vi "GUI_laptop v8.vi"() -> ()   [LabVIEW 2019]
uses:
  <vilib>/Math Plots/3D Math Plots/3D Scatter/3D Scatter XCtrl/3D Scatter.xctl
  <vilib>/Platform/TimedLoop/XDataNode/timing_clust.ctl
  <vilib>/Platform/TimedLoop/XDataNode/nitl_modes.ctl
  <vilib>/Platform/TimedLoop/XDataNode/wakeup.ctl
  <vilib>/Analysis/_algsub.llb/Real Vector Norm.vi
  <vilib>/Instr/_visa.llb/VISA Configure Serial Port (Instr).vi
  <vilib>/Utility/file.llb/Write Delimited Spreadsheet (DBL).vi
  <vilib>/Math Plots/3D Math Plots/3D Scatter/3D Scatter Datatype/Public/Plot Helper (Vector).vi
  <vilib>/platform/TimedLoop/XDataNode/XDataNode.xnode
  <vilib>/Platform/TimedLoop/XDataNode/XDNodeRunTimeDep.lvlib
  <vilib>/Analysis/NI_AALPro.lvlib
  <vilib>/Math Plots/3D Math Plots/3D Scatter/3D Scatter Datatype/3D Scatter Datatype.lvclass
panel:
  out "send values":dbl[](array[numeric])
  out "Robot Feedback (xyz)":dbl[](array[numeric])
  in  "UDP Send":bool
  in  "UDP Recv":bool
  in  "L5 bound":dbl=1000.0
  in  "L4 bound (deg)":dbl=1000.0
  in  "L3 bound (mm)":dbl=1000.0
  in  "L2 bound (deg)":dbl=1000.0
  in  "L1 bound (deg)":dbl=1000.0
  in  "Joystick Type":dbl(ring) items=["Rigid Joystick", "Free Joystick"]
  out "Finished Late? [i-1]":bool
  in  "Epsilon":dbl=0.2
  out "3D Scatter":refnum<class "3D Plot Datatype.lvclass">[](xcontrol)
  out "Random Point":dbl[](array[numeric])
  out "Virtual Cursor":dbl[](array[numeric])
  out "Iteration Duration":i64
  in  "Num of Points":i32=10
  in  "z bound":dbl=2.0
  in  "y bound":dbl=5.0
  in  "x bound":dbl=5.0
  in  "Stop":bool
  in  "Round Decimals":dbl=2.0 format="%#_15g"
  in  "Save  Data":bool
  in  "Save Path":path
  in  "x speed":dbl=0.5
  in  "z speed":dbl=0.5
  in  "y speed":dbl=0.5
  out "error out":errorcluster
  in  "baud rate":u32=115200
  in  "VISA resource name":refnum<visa-resource-name>
  # "TODO: fix the bounds; currently bounds are arbitrary"
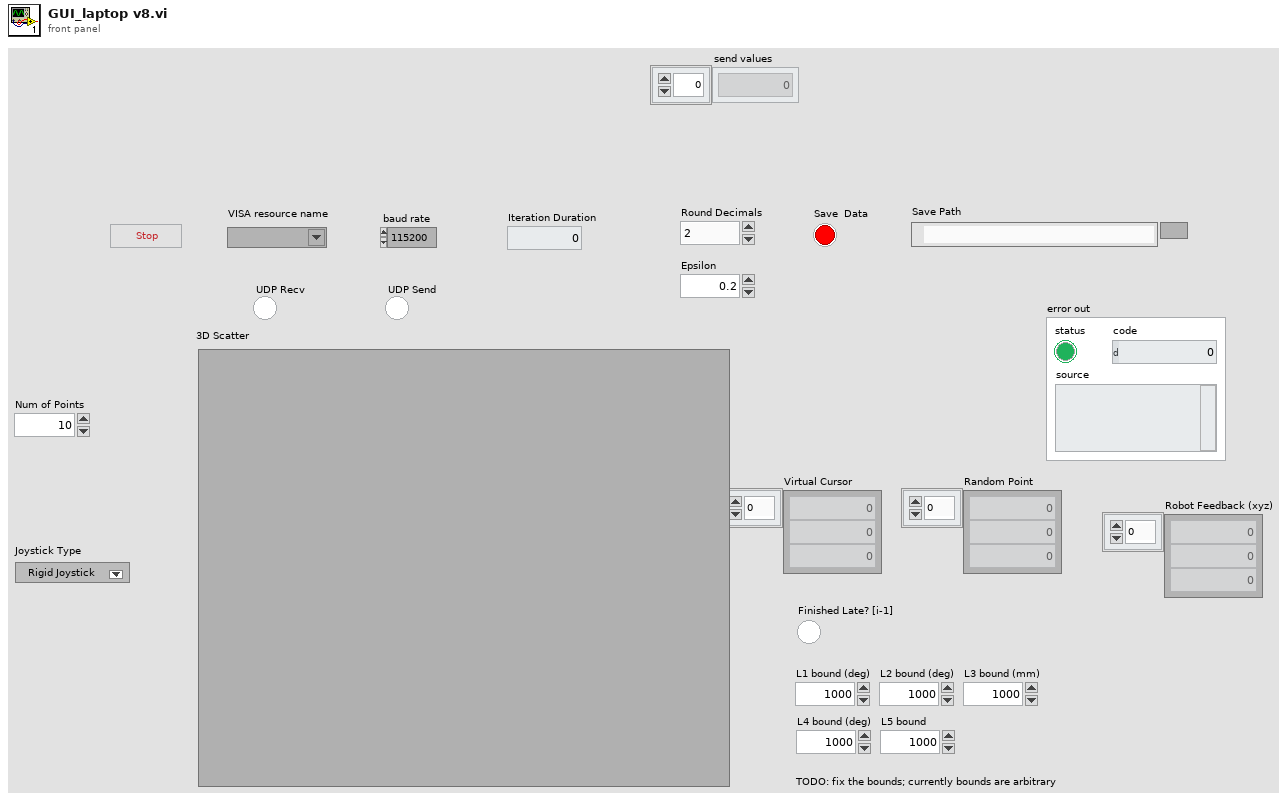
[diagram p1: front panel]
types:
  T1 = typedef "XDNodeRunTimeDep.lvlib/timing_clust.ctl" = cluster{"Expected End [f-1]":u64, "Actual End [f-1]":u64, "Finished Late? [f-1]":bool, "Expected End [i-1]":u64, "Actual End [i-1]":u64, "Finished Late? [i-1]":bool, "Expected Start [i]":u64, "Actual Start [i]":u64, "Expected Start [f]":u64, "Actual Start [f]":u64, "Source Name":string, "Structure Name":string, "Period":i64, "Deadline":i64, "Offset":i64, "Start":i64, "Priority":i32, "Timeout":i32, "Mode":T2, "Wakeup Reason":T3, "Error":errorcluster, "Source Type":string, "Secondary Source Type":string, "Global End Time":u64, "Global Start Time":u64, "Frame Duration":u64, "Iteration Duration":u64, "Assigned CPU":i32, "I/O Scan Engine Mode":u32}
  T2 = typedef "XDNodeRunTimeDep.lvlib/nitl_modes.ctl" = enum32{"No Change", "Process missed periods, maintain original phase", "Discard missed periods, maintain original phase", "Process missed periods, ignore original phase", "Discard missed periods, ignore original phase"}
  T3 = typedef "XDNodeRunTimeDep.lvlib/wakeup.ctl" = enum32{"Normal", "Aborted", "Asynchronous wakeup", "Timing source error", "Timed loop error", "Timeout"}
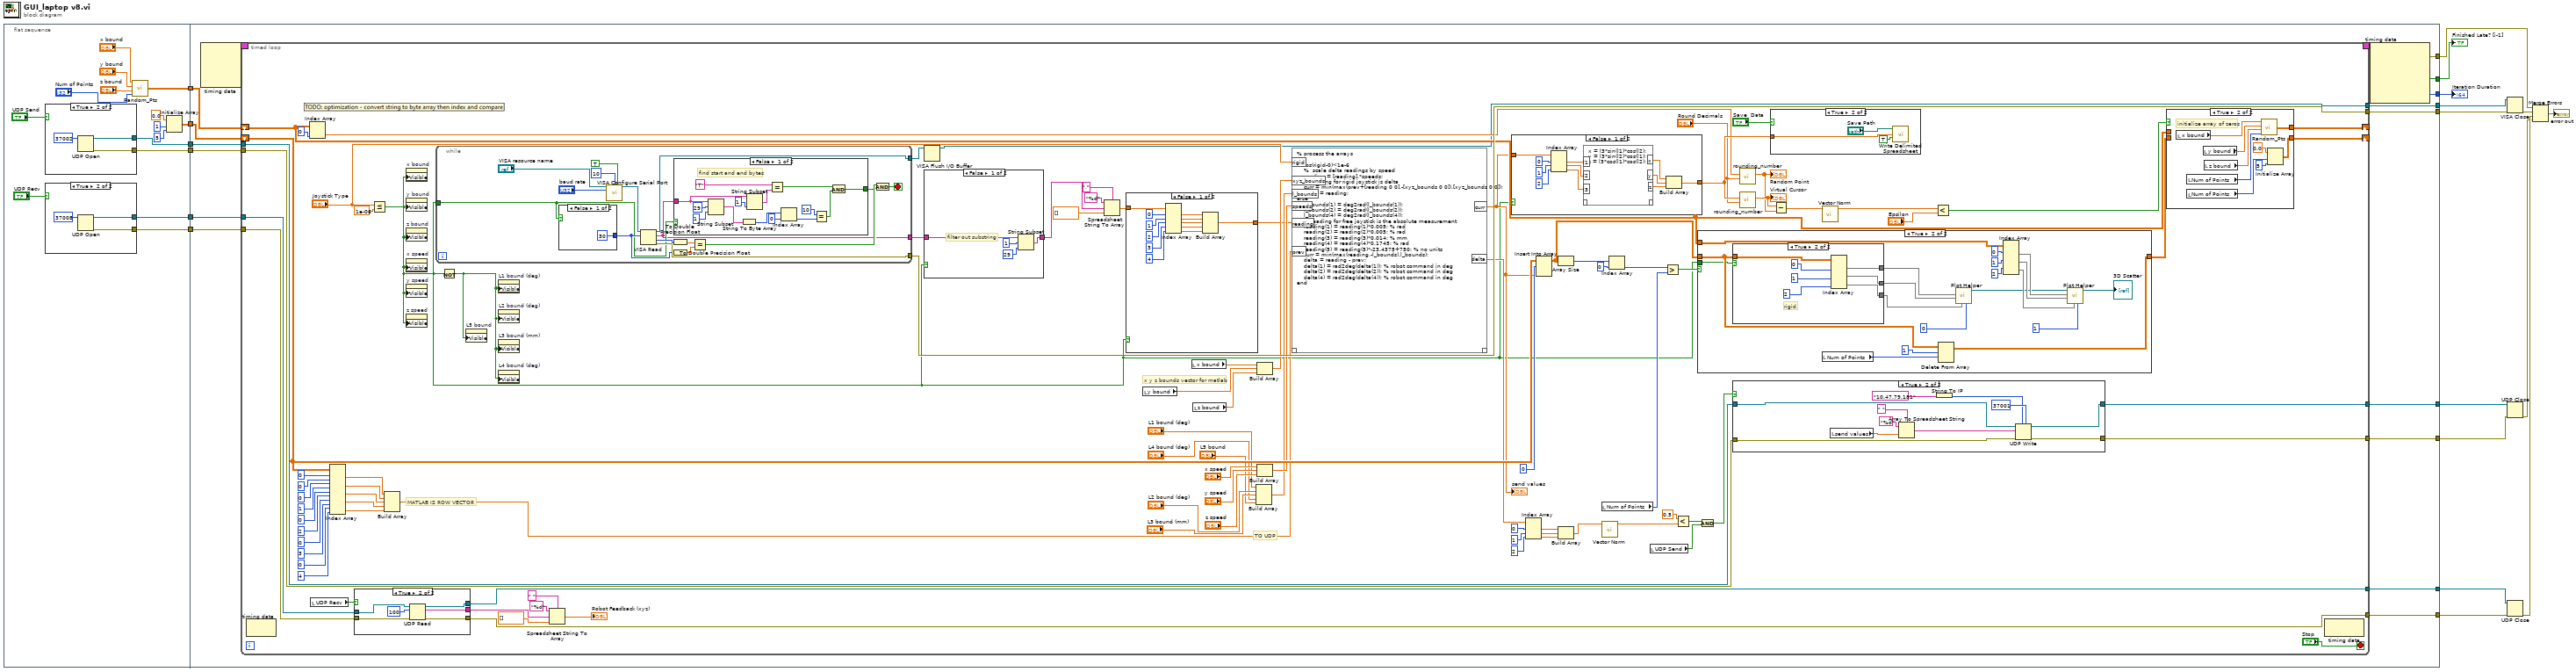
[diagram p0: block diagram]
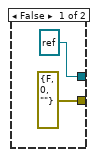
[diagram p2: hidden frame]
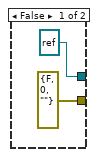
[diagram p3: hidden frame]
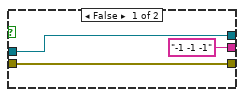
[diagram p5: hidden frame]
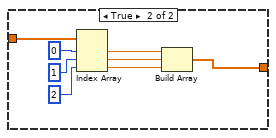
[diagram p9: hidden frame]
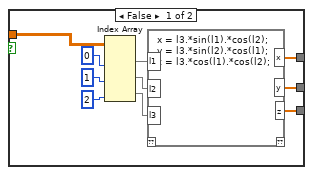
[diagram p12: hidden frame]
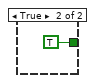
[diagram p13: hidden frame]
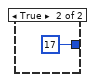
[diagram p14: hidden frame]
diagram:
  n1 = flat-sequence {
    tunnel: [w26] -> w15
    tunnel: [w30] -> w14
    tunnel: [w25] -> w13
    tunnel: [w24] -> w12
    tunnel: [w21] -> w11
    tunnel: [w20] -> w10
    tunnel: [w59] -> w19
    tunnel: [w58] -> w18
    tunnel: [w56] -> w9
    tunnel: [w54] -> w17
    tunnel: [w53] -> w16
    tunnel: w15 -> [w57]
    tunnel: w14 -> [w55]
    tunnel: w13 -> [w52]
    tunnel: w12 -> [w51]
    tunnel: w11 -> [w50]
    tunnel: w10 -> [w49]
    tunnel: [w48] -> w3
    tunnel: [w47] -> w8
    tunnel: [w46] -> w2
    tunnel: [w45] -> w1
    frame #0 {
      n2 = case shown="True" "UDP Send" {
        tunnel: [refnum<k16> refnum ("port") w38] -> w25
        tunnel: [errorcluster {"status"=FALSE, "code"=0, "source"=""} ("error out") w37] -> w20
        frame False {
        }
        frame True {
          n3 = UDP Open(11:u16 37002 ("port")) -> (port=w38:refnum<k16>, 0:w37:errorcluster)  [unwired: 4 in, 1 out]
        }
      }
      n4 = case shown="True" "UDP Recv" {
        tunnel: [refnum<k16> refnum ("port") w43] -> w24
        tunnel: [errorcluster {"status"=FALSE, "code"=0, "source"=""} ("error out") w42] -> w21
        frame False {
        }
        frame True {
          n5 = UDP Open(11:u16 37008 ("port")) -> (port=w43:refnum<k16>, 0:w42:errorcluster)  [unwired: 4 in, 1 out]
        }
      }
      n6 = call "Random_Pts.vi"("Num of Points"="Num of Points", "z bound"="z bound", "y bound"="y bound", "x bound"="x bound") -> ("appended array"=w30:dbl[][])
      n7 = Initialize Array(0.0 ("element"), 1 ("dimension size"), 5 ("dimension size")) -> (w26:dbl[][])
    }
    frame #1 {
      n8 = node-c288() -> (w61:T1)  [unwired: 4 in]
      n9 = timed-loop {
        tunnel: [w92] -> w59
        tunnel: [w156] -> w58
        shift-right: [w155] -> _
        shift-left: w57 -> [w154]
        timing: w61 -> [_]
        timing-out: [_] -> w60
        shift-right: [w150] -> _
        shift-left: w55 -> [w151]
        tunnel: w52 -> [w91]
        tunnel: w51 -> [w90]
        tunnel: w50 -> [w88]
        tunnel: w49 -> [w87]
        tunnel: [w86] -> w48
        tunnel: [w85] -> w47
        tunnel: [w84] -> w46
        tunnel: [w83] -> w45
        stop <- "Stop" stop-if-true
        # "TO UDP"
        # "MATLAB IS ROW VECTOR"
        # "x y z bounds vector for matlab"
        n10 = node-c288() -> ()  [unwired: 1 in, 1 out]
        n11 = Index Array(array=w151, index (col)=0 ("index (row)")) -> (element=w103:dbl[])  [unwired: 1 in]
        n12 = local read "UDP Recv"() -> (w89:bool)
        n13 = Index Array(array=w154, index (row) #1=0 ("disabled index (row)"), index (col) #1=0 ("disabled index (col)"), index (row) #2=0 ("disabled index (row)"), index (col) #2=1 ("disabled index (col)"), index (row) #3=0 ("disabled index (row)"), index (col) #3=2 ("disabled index (col)"), index (row) #4=0 ("disabled index (row)"), index (col) #4=3 ("disabled index (col)"), index (row) #5=0 ("disabled index (row)"), index (col) #5=4 ("disabled index (col)")) -> (element #1=w127:dbl, element #2=w126:dbl, element #3=w125:dbl, element #4=w111:dbl, element #5=w110:dbl)
        n14 = case shown="True" w89 {
          tunnel: w90 -> [w172 w179]
          tunnel: w88 -> [w173 w178]
          tunnel: [w173 w177] -> w86
          tunnel: [w172 w176] -> w84
          tunnel: ["-1 -1 -1" w174] -> w79
          frame False {
          }
          frame True {
            n15 = UDP Read(connection ID=w179, max size (548)=100, 8:w178) -> (data out=w174:string, error out=w177:errorcluster, 3:w176:refnum<k16>)  [unwired: 1 in, 2 out]
          }
        }
        n16 = Less Or Equal?(x="Joystick Type", y=1e-06) -> (x <= y?=w63:bool)
        n17 = Build Array(w127, w126, w125, w111, w110) -> (w124:dbl[])
        n18 = property on="x bound" class="DigNum (strict)"("Visible"=w63) -> ()  [unwired: 2 in, 2 out]
        n19 = property on="y bound" class="DigNum (strict)"("Visible"=w63) -> ()  [unwired: 2 in, 2 out]
        n20 = property on="z bound" class="DigNum (strict)"("Visible"=w63) -> ()  [unwired: 2 in, 2 out]
        n21 = property on="x speed" class="DigNum (strict)"("Visible"=w63) -> ()  [unwired: 2 in, 2 out]
        n22 = property on="y speed" class="DigNum (strict)"("Visible"=w63) -> ()  [unwired: 2 in, 2 out]
        n23 = property on="z speed" class="DigNum (strict)"("Visible"=w63) -> ()  [unwired: 2 in, 2 out]
        n24 = while {
          tunnel: [w268] -> w105
          tunnel: [w281] -> w156
          tunnel: [w275] -> w93
          tunnel: w63 -> [w269]
          stop <- w271 stop-if-true
          n25 = case shown="False" w269 {
            tunnel: [30 u32 17 ("byte count")] -> w274
            frame False {
            }
            frame True {
            }
          }
          n26 = call-poly "VISA Configure Serial Port"("VISA resource name"="VISA resource name", "termination char\n(0xA = '\\n' = LF)"=u8 10 ("termination char\n(0xA = '\\n' = LF)"), "Enable Termination\nChar (T)"=TRUE ("Enable Termination\nChar (T)"), "baud rate (9600)"="baud rate") -> ("VISA resource name out"=w276:refnum<visa-resource-name>)  [unwired: 10 in, 1 out]
          n27 = VISA Read(VISA resource name=w276, byte count=w274) -> (VISA resource name out=w275:refnum<visa-resource-name>, read buffer=w268:string, return count=w283:u32, error out=w281:errorcluster)  [unwired: 1 in]
          n28 = To Double Precision Float(number=w283) -> (double precision float=w282:dbl)
          n29 = To Double Precision Float(number=w274) -> (double precision float=w273:dbl)
          n30 = case shown="False" w269 {
            tunnel: [w290 TRUE] -> w270
            tunnel: w268 -> [w293 _]
            frame False {
              # "find start and end bytes"
              n31 = String Subset(string=w293, offset (0)=29, length (rest)=1) -> (substring=w288:string)
              n32 = String To Byte Array(string=w288) -> (unsigned byte array=w287:u8[])
              n33 = String Subset(string=w293, length (rest)=1) -> (substring=w296:string)  [unwired: 1 in]
              n34 = Equal?(x="T", y=w296) -> (x = y?=w292:bool)
              n35 = Index Array(array=w287, index=0) -> (element=w285:u8)
              n36 = Equal?(x=10, y=w285) -> (x = y?=w291:bool)
              n37 = And(x=w292, y=w291) -> (x .and. y?=w290:bool)
            }
            frame True {
            }
          }
          n38 = Equal?(x=w282, y=w273) -> (x = y?=w272:bool)
          n39 = And(x=w272, y=w270) -> (x .and. y?=w271:bool)
        }
        n40 = Not(x=w63) -> (.not. x?=w62:bool)
        n41 = property on="L5 bound" class="DigNum (strict)"("Visible"=w62) -> ()  [unwired: 2 in, 2 out]
        n42 = property on="L1 bound (deg)" class="DigNum (strict)"("Visible"=w62) -> ()  [unwired: 2 in, 2 out]
        n43 = property on="L2 bound (deg)" class="DigNum (strict)"("Visible"=w62) -> ()  [unwired: 2 in, 2 out]
        n44 = property on="L3 bound (mm)" class="DigNum (strict)"("Visible"=w62) -> ()  [unwired: 2 in, 2 out]
        n45 = property on="L4 bound (deg)" class="DigNum (strict)"("Visible"=w62) -> ()  [unwired: 2 in, 2 out]
        n46 = Spreadsheet String To Array(delimiter (Tab)=" ", format string="%d", spreadsheet string=w79, array type (2D Dbl)=dbl[] []) -> (array=→"Robot Feedback (xyz)":dbl[])
        n47 = VISA Flush I/O Buffer(VISA resource name=w93) -> (VISA resource name out=w92:refnum<visa-resource-name>)  [unwired: 2 in, 1 out]
        n48 = case shown="False" w63 {
          tunnel: w105 -> [w197 w198]
          tunnel: [w194 w198] -> w104
          frame False {
            # "filter out substring"
            n49 = String Subset(string=w197, offset (0)=1, length (rest)=29) -> (substring=w194:string)
          }
          frame True {
          }
        }
        n50 = Spreadsheet String To Array(delimiter (Tab)=",", format string="%d", spreadsheet string=w104, array type (2D Dbl)=dbl[] []) -> (array=w107:dbl[])
        n51 = case shown="False" w63 {
          tunnel: w107 -> [w199 w212]
          tunnel: [w204 w211] -> w106
          frame False {
            n52 = Index Array(array=w199, index #1=0 ("Plot ID"), index #2=1 ("Plot ID"), index #3=2 ("Plot ID"), index #4=3 ("Plot ID"), index #5=4 ("Plot ID")) -> (element #1=w207:dbl, element #2=w206:dbl, element #3=w205:dbl, element #4=w201:dbl, element #5=w200:dbl)
            n53 = Build Array(w207, w206, w205, w201, w200) -> (w204:dbl[])
          }
          frame True {
            n54 = Index Array(array=w212, index #1=0 ("Plot ID"), index #2=1 ("Plot ID"), index #3=2 ("Plot ID")) -> (element #1=w215:dbl, element #2=w214:dbl, element #3=w213:dbl)
            n55 = Build Array(w215, w214, w213) -> (w211:dbl[])
          }
        }
        n56 = local read "y bound"() -> (w129:dbl)
        n57 = local read "x bound"() -> (w130:dbl)
        n58 = local read "z bound"() -> (w128:dbl)
        n59 = Build Array("L1 bound (deg)", "L2 bound (deg)", "L3 bound (mm)", "L4 bound (deg)", "L5 bound") -> (w118:dbl[])
        n60 = Build Array(w130, w129, w128) -> (w122:dbl[])
        n61 = Build Array("x speed", "y speed", "z speed") -> (w123:dbl[])
        n62 = script code="% process the arrays\n\nif abs(rigid-0)<1e-6\n    %  scale delta readings by speed\n    reading = [reading].*speeds;\n    % reading for rigid joystick is delta\n    curr = min(max(prev+[reading 0 0],-[xyz_bounds 0 0]),[xyz_bounds 0 0]);\n    delta = reading;\nelse\n    l_bounds(1) = deg2rad(l_bounds(1));\n    l_bounds(2) = deg2rad(l_bounds(2));\n    l_bounds(4) = deg2rad(l_bounds(4));\n    % reading for free joystick is the absolute measurement\n    reading(1) = reading(1)*0.005; % rad\n    reading(2) = reading(2)*0.005; % rad\n    reading(3) = reading(3)*0.014; % mm\n    reading(4) = reading(4)*0.1745; % rad\n    reading(5) = reading(5)*-23.4375+750; % no units\n    curr = min(max(reading,-l_bounds),l_bounds);\n    delta = reading - prev;\n    delta(1) = rad2deg(delta(1)); % robot command in deg\n    delta(2) = rad2deg(delta(2)); % robot command in deg\n    delta(4) = rad2deg(delta(4)); % robot command in deg\nend"("xyz_bounds"=w122, "speeds"=w123, "reading"=w106, "prev"=w124, "rigid"="Joystick Type", "l_bounds"=w118) -> ("curr"=w64:dbl[], "delta"=w72:dbl[])  [unwired: 1 in, 1 out]
        "send values" <- w64
        n63 = case shown="False" w63 {
          tunnel: w64 -> [w226 w230]
          tunnel: [w219 w230] -> w152
          frame False {
            n64 = Index Array(array=w226, index #1=0 ("Plot ID"), index #2=1 ("Plot ID"), index #3=2 ("Plot ID")) -> (element #1=w225:dbl, element #2=w224:dbl, element #3=w223:dbl)
            n65 = script code="x = l3*sin(l1)*cos(l2);\ny = l3*sin(l2)*cos(l1);\nz = l3*cos(l1)*cos(l2);"("l1"=w225, "l2"=w224, "l3"=w223) -> ("x"=w222:dbl, "y"=w221:dbl, "z"=w220:dbl)  [unwired: 1 in, 1 out]
            n66 = Build Array(w222, w221, w220) -> (w219:dbl[])
          }
          frame True {
          }
        }
        n67 = Index Array(array=w72, index #1=0 ("disabled index (col)"), index #2=1 ("disabled index (col)"), index #3=2 ("disabled index (col)")) -> (element #1=w68:dbl, element #2=w67:dbl, element #3=w66:dbl)
        n68 = Insert Into Array(array=w154, index (row)=0, new element=w64) -> (w135:dbl[][])  [unwired: 1 in]
        n69 = Array Size(array=w135) -> (size(s)=w137:i32[])
        n70 = Build Array(w68, w67, w66) -> (w65:dbl[])
        n71 = local read "Num of Points"() -> (w136:i32)
        n72 = call-poly <vilib>:"Vector Norm.vi"("Input Vector"=w65) -> ("norm"=w77:dbl)  [unwired: 9 in, 1 out]
        n73 = Index Array(array=w137, index=0) -> (element=w138:i32)
        n74 = local read "UDP Send"() -> (w74:bool)
        n75 = Greater?(x=w138, y=w136) -> (0:w134:bool)
        n76 = Less?(x=0.5, y=w77) -> (x < y?=w75:bool)
        n77 = case shown="True" w134 {
          tunnel: w135 -> [w231 w249]
          tunnel: [w231 w248] -> w153
          tunnel: w151 -> [_ w247]
          tunnel: w63 -> [_ w232]
          frame False {
          }
          frame True {
            n78 = case shown="True" w232 {
              tunnel: w249 -> [w260 w264]
              tunnel: [w251 w263] -> w238
              tunnel: [w252 w262] -> w237
              tunnel: [w253 w261] -> w236
              frame False {
                n79 = Index Array(array=w260, index (col) #1=0 ("Plot ID"), index (col) #2=1 ("Plot ID"), index (col) #3=2 ("Plot ID")) -> (element #1=w256:dbl[], element #2=w255:dbl[], element #3=w254:dbl[])  [unwired: 3 in]
                n80 = script code="x = l3.*sin(l1).*cos(l2);\ny = l3.*sin(l2).*cos(l1);\nz = l3.*cos(l1).*cos(l2);"("l1"=w256, "l2"=w255, "l3"=w254) -> ("x"=w251:dbl[], "y"=w252:dbl[], "z"=w253:dbl[])  [unwired: 1 in, 1 out]
              }
              frame True {
                # "rigid"
                n81 = Index Array(array=w264, index (col) #1=0 ("disabled index (col)"), index (col) #2=1 ("index (col)"), index (col) #3=2 ("index (col)")) -> (element #1=w263:dbl[], element #2=w262:dbl[], element #3=w261:dbl[])  [unwired: 3 in]
              }
            }
            n82 = local read "Num of Points"() -> (w246:i32)
            n83 = Delete From Array(array=w249, length=1, index (row)=w246) -> (array with subset deleted=w248:dbl[][])  [unwired: 1 in, 1 out]
            n84 = call-poly <vilib>:"Plot Helper.vi"("Plot ID"=0, "z vector"=w236, "y vector"=w237, "x vector"=w238) -> ("3D Plot lvclass Array out"=w240:refnum<class "3D Plot Datatype.lvclass">[])  [unwired: 2 in, 5 out]
            n85 = Index Array(array=w247, index (row) #1=0 ("index (row)"), index (row) #2=1 ("index (row)"), index (row) #3=2 ("index (row)")) -> (element #1=w244:dbl[], element #2=w243:dbl[], element #3=w242:dbl[])  [unwired: 3 in]
            n86 = call-poly <vilib>:"Plot Helper.vi"("Plot ID"=1, "z vector"=w242, "y vector"=w243, "x vector"=w244, "3D Plot lvclass Array in"=w240) -> ("3D Plot lvclass Array out"=→"3D Scatter":refnum<class "3D Plot Datatype.lvclass">[])  [unwired: 1 in, 5 out]
          }
        }
        n87 = And(x=w75, y=w74) -> (x .and. y?=w73:bool)
        n88 = case shown="True" w73 {
          tunnel: w91 -> [w158 w170]
          tunnel: w87 -> [w159 w166]
          tunnel: [w159 w162] -> w85
          tunnel: [w158 w161] -> w83
          frame False {
          }
          frame True {
            n89 = local read "send values"() -> (w160:dbl[])
            n90 = Array To Spreadsheet String(delimiter (Tab)=" ", array=w160, 3:"%d" ("format string")) -> (spreadsheet string=w167:string)
            n91 = String To IP(1:"10.47.79.181" ("name")) -> (0:w164:u32)
            n92 = UDP Write(address=w164, port or service name=u16 37001, connection ID=w170, data in=w167, 8:w166) -> (error out=w162:errorcluster, 3:w161:refnum<k16>)  [unwired: 1 in]
          }
        }
        n93 = call "rounding_number.vi"("power of ten"="Round Decimals", "Array"=w103) -> ("rounded"=w99:dbl[])  [unwired: 9 in]
        "Random Point" <- w99
        n94 = call "rounding_number.vi"("power of ten"="Round Decimals", "Array"=w152) -> ("rounded"=w100:dbl[])  [unwired: 9 in]
        "Virtual Cursor" <- w100
        n95 = case shown="True" "Save  Data" {
          tunnel: w152 -> [_ w180]
          frame False {
          }
          frame True {
            n96 = call-poly <vilib>:"Write Delimited Spreadsheet.vi"("file path (dialog if empty)"="Save Path", "1D data"=w180, "append to file? (new file:F)"=TRUE) -> ()  [unwired: 11 in, 2 out]
          }
        }
        n97 = Subtract(x=w100, y=w99) -> (x-y=w98:dbl[])
        n98 = call-poly <vilib>:"Vector Norm.vi"("Input Vector"=w98) -> ("norm"=w97:dbl)  [unwired: 9 in, 1 out]
        n99 = Less?(x=w97, y="Epsilon") -> (x < y?=w95:bool)
        n100 = case shown="True" w95 {
          tunnel: w151 -> [w184 _]
          tunnel: [w184 w189] -> w150
          tunnel: w153 -> [w183 _]
          tunnel: [w183 w185] -> w155
          frame False {
          }
          frame True {
            # "initialize array of zeros"
            n101 = local read "x bound"() -> (w193:dbl)
            n102 = local read "Num of Points"() -> (w190:i32)
            n103 = local read "Num of Points"() -> (w187:i32)
            n104 = local read "y bound"() -> (w192:dbl)
            n105 = local read "z bound"() -> (w191:dbl)
            n106 = call "Random_Pts.vi"("Num of Points"=w190, "z bound"=w191, "y bound"=w192, "x bound"=w193) -> ("appended array"=w189:dbl[][])
            n107 = Initialize Array(0.0 ("element"), w187, 5 ("dimension size")) -> (w185:dbl[][])
          }
        }
        n108 = node-c288() -> ()  [unwired: 1 in, 1 out]
      }
      n109 = node-c288(w60) -> (w56:errorcluster, w53:bool, w54:i64)  [unwired: 3 out]
    }
  }
  n110 = VISA Close(VISA resource name=w19, error in (no error)=w18) -> (error out=w7:errorcluster)
  n111 = UDP Close(connection ID=w1, 8:w8) -> (error out=w5:errorcluster)  [unwired: 1 out]
  n112 = UDP Close(connection ID=w2, 8:w3) -> (error out=w6:errorcluster)  [unwired: 1 out]
  n113 = Merge Errors(w9, w7, w6, w5) -> (→"error out":errorcluster)
  "Iteration Duration" <- w17
  "Finished Late? [i-1]" <- w16
